vi "Write--command.vi"(8 "error in (no error)":errorcluster, 10 "Command":string, 11 "VISA resource name":refnum<visa-resource-name>) -> (0 "error out":errorcluster, 2 "Command out":string, 3 "VISA resource name out":refnum<visa-resource-name>)   [LabVIEW 2025, in "Control de MaP.lvlib"]
doc: "convierte la selección de comando a cadena y lo envía al puerto seleccionado"
uses:
  Control de MaP.lvlib
  <vilib>/Instr/_visa.llb/VISA Flush IO Buffer Mask.ctl
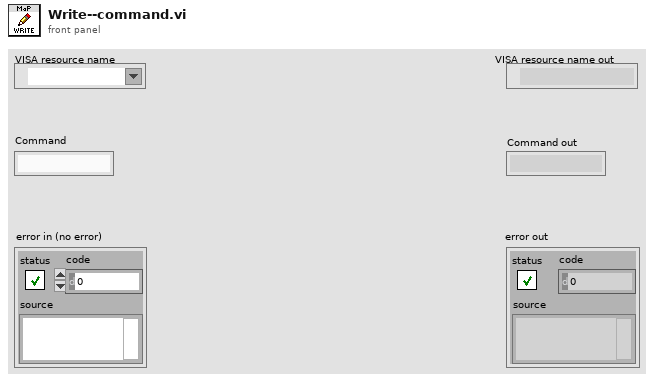
[diagram p1: front panel]
types:
  T1 = typedef "VISA Flush IO Buffer Mask.ctl" = u16
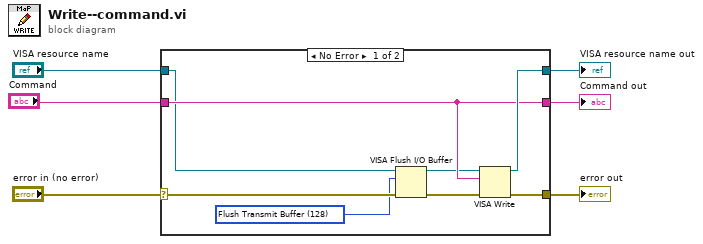
[diagram p0: block diagram]
diagram:
  n1 = case shown="No Error" "error in (no error)" {
    selector: "error in (no error)" -> [w11 w16]
    tunnel: "VISA resource name" -> [w9 w15]
    tunnel: [w14 w15] -> w5
    tunnel: [w13 w16] -> w3
    tunnel: "Command" -> [w12 _]
    tunnel: [w12 _] -> w1
    frame No Error {
      w7 = T1 128 items=["Flush Receive Buffer"=16, "Write Transmit Buffer to Device"=32, "Flush Receive Buffer (No I/O)"=64, "Flush Transmit Buffer"=128] ("Mask")
      n2 = VISA Flush I/O Buffer(VISA resource name=w9, mask (16)=w7, error in (no error)=w11) -> (VISA resource name out=w8:refnum<visa-resource-name>, error out=w10:errorcluster)
      n3 = VISA Write(VISA resource name=w8, write buffer=w12, error in (no error)=w10) -> (VISA resource name out=w14:refnum<visa-resource-name>, error out=w13:errorcluster)  [unwired: 1 out]
    }
    frame Error {
    }
  }
  "VISA resource name out" <- w5
  "error out" <- w3
  "Command out" <- w1
